vi "GearRectangleCompare.vi"(6 "Line Border":cluster{"Top":dbl, "Bottom":dbl}={"Top"=6.0, "Bottom"=1.0}, 9 "Second":dbl[](array[numeric]), 11 "First":dbl[](array[numeric])) -> (0 "Rect":T1, 1 "Line":T1, 3 "Scores":T2)   [LabVIEW 2016]
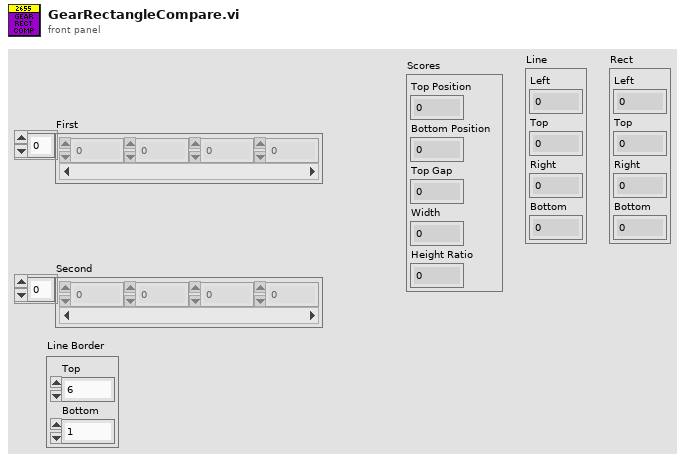
[diagram p1: front panel]
types:
  T1 = cluster{"Left":dbl, "Top":dbl, "Right":dbl, "Bottom":dbl}
  T2 = cluster{"Top Position":dbl, "Bottom Position":dbl, "Top Gap":dbl, "Width":dbl, "Height Ratio":dbl}
  T3 = cluster{"Top Position":dbl, "Bottom Position":dbl, "Left Gap":dbl, "Width":dbl}
  T4 = cluster{"Top Position":dbl, "Bottom Position":dbl, "Left Gap":dbl, "Width":dbl, "Height Ratio":dbl}
  T5 = cluster{"[0]":dbl, "[1]":dbl, "[2]":dbl, "[3]":dbl}
  T6 = cluster{"Top Position":dbl, "Top Position":dbl, "Top Position":dbl, "Top Position":dbl}
  T7 = cluster{"upper limit":dbl, "upper limit":dbl, "upper limit":dbl, "upper limit":dbl, "upper limit":dbl}
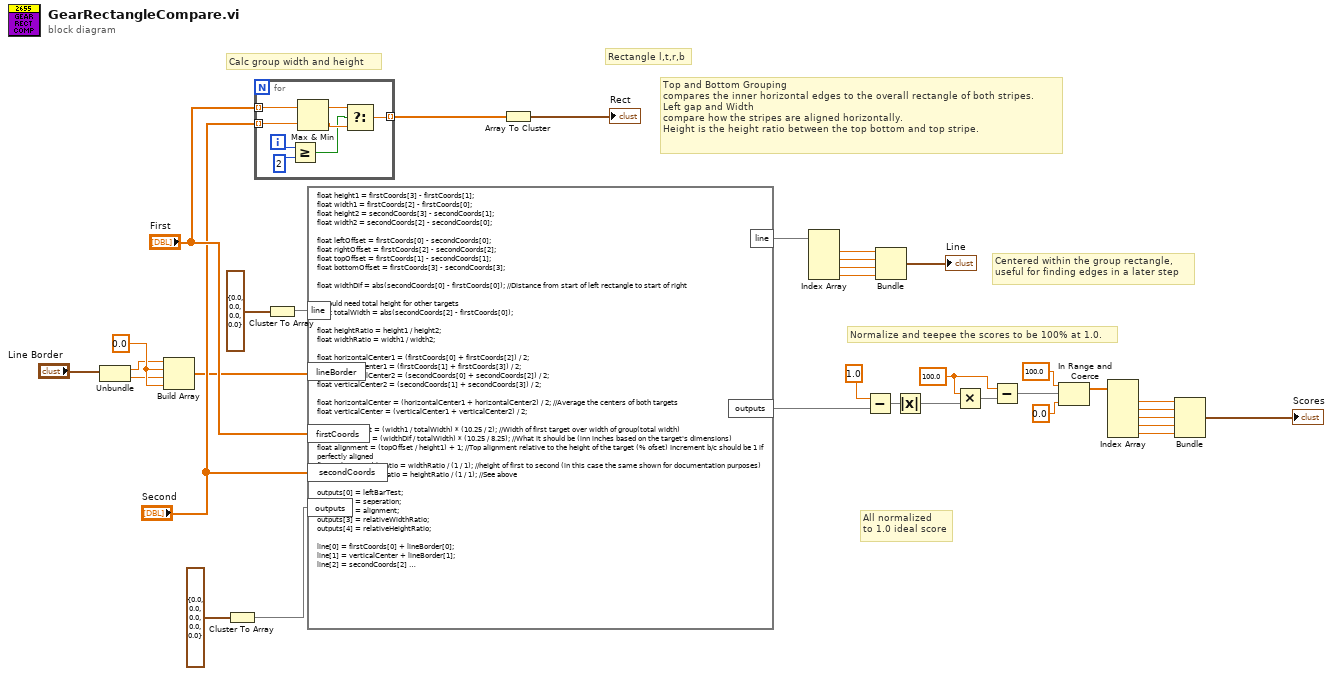
[diagram p0: block diagram]
diagram:
  w3 = 0.0 ("element")
  w31 = 100.0 ("x/y")
  # "Centered within the group rectangle,\nuseful for finding edges in a later step"
  # "All normalized\nto 1.0 ideal score"
  # "Normalize and teepee the scores to be 100% at 1.0."
  # "Top and Bottom Grouping\ncompares the inner horizontal edges to the overall rectangle of both stripes.\nLeft gap and Width\ncompare how the stripes are aligned horizontally.\nHeight is the height ratio between the top bottom and top stripe."
  # "Calc group width and height"
  # "Rectangle l,t,r,b"
  n1 = Unbundle("Line Border") -> ("Top"=w2:dbl, "Bottom"=w1:dbl)
  n2 = Build Array(w2, w3, w1, w3) -> (w4:dbl[])
  n3 = Cluster To Array(cluster=T4 {"Top Position"=0.0, "Bottom Position"=0.0, "Left Gap"=0.0, "Width"=0.0, "Height Ratio"=0.0} ("Scores 2")) -> (array=w14:dbl[])
  n4 = for {
    tunnel: "First" -> [w43] mode=indexing
    tunnel: "Second" -> [w42] mode=indexing
    tunnel: [w36] -> w35 mode=indexing
    i -> [w40]
    n5 = Greater Or Equal?(x=w40, y=2) -> (x >= y?=w37:bool)
    n6 = Max & Min(x=w43, y=w42) -> (max(x,y)=w39:dbl, min(x,y)=w38:dbl)
    n7 = Select(t=w39, s=w37, f=w38) -> (s? t:f=w36:dbl)
  }
  n8 = Cluster To Array(cluster=T3 {"Top Position"=0.0, "Bottom Position"=0.0, "Left Gap"=0.0, "Width"=0.0} ("Scores 2")) -> (array=w12:dbl[])
  n9 = formula code="float height1 = firstCoords[3] - firstCoords[1];\nfloat width1 = firstCoords[2] - firstCoords[0];\nfloat height2 = secondCoords[3] - secondCoords[1];\nfloat width2 = secondCoords[2] - secondCoords[0];\n\nfloat leftOffset = firstCoords[0] - secondCoords[0];\nfloat rightOffset = firstCoords[2] - secondCoords[2];\nfloat topOffset = firstCoords[1] - secondCoords[1];\nfloat bottomOffset = firstCoords[3] - secondCoords[3];\n\t\nfloat widthDif = abs(secondCoords[0] - firstCoords[0]); //Distance from start of left rectangle to start of right\n\t\n//Would need total height for other targets\nfloat totalWidth = abs(secondCoords[2] - firstCoords[0]);\n\t\nfloat heightRatio = height1 / height2;\nfloat widthRatio = width1 / width2;\n\nfloat horizontalCenter1 = (firstCoords[0] + firstCoords[2]) / 2;\nfloat verticalCenter1 = (firstCoords[1] + firstCoords[3]) / 2;\nfloat horizontalCenter2 = (secondCoords[0] + secondCoords[2]) / 2;\nfloat verticalCenter2 = (secondCoords[1] + secondCoords[3]) / 2;\n\nfloat horizontalCenter = (horizontalCenter1 + horizontalCenter2) / 2; //Average the centers of both targets\nfloat verticalCenter = (verticalCenter1 + verticalCenter2) / 2;\n\t\t\nfloat leftBarTest = (width1 / totalWidth) * (10.25 / 2); //Width of first target over width of group(total width)\nfloat seperation = (widthDif / totalWidth) * (10.25 / 8.25); //What it should be (inn inches based on the target's dimensions)\nfloat alignment = (topOffset / height1) + 1; //Top alignment relative to the height of the target (% ofset) Increment b/c should be 1 if perfectly aligned\nfloat relativeWidthRatio = widthRatio / (1 / 1); //height of first to second (in this case the same shown for documentation purposes)\nfloat relativeHeightRatio = heightRatio / (1 / 1); //See above\n\t\t\t\t\noutputs[0] = leftBarTest;\noutputs[1] = seperation;\noutputs[2] = alignment;\noutputs[3] = relativeWidthRatio;\noutputs[4] = relativeHeightRatio;\n\t\t\nline[0] = firstCoords[0] + lineBorder[0];\nline[1] = verticalCenter + lineBorder[1];\nline[2] = secondCoords[2] - lineBorder[2];\nline[3] = verticalCenter - lineBorder[3];"("firstCoords"="First", "secondCoords"="Second", "outputs"=w14, "line"=w12, "lineBorder"=w4) -> ("outputs"=w23:dbl[], "line"=w7:dbl[])
  n10 = Array To Cluster(array=w35) -> (cluster=→"Rect":T5)
  n11 = Index Array(array=w7) -> (element #1=w11:dbl, element #2=w10:dbl, element #3=w9:dbl, element #4=w8:dbl)  [unwired: 4 in]
  n12 = Subtract(x=1.0 ("y"), y=w23) -> (x-y=w29:dbl[])
  n13 = Bundle("Top Position"=w11, "Top Position"=w10, "Top Position"=w9, "Top Position"=w8) -> (→"Line":T6)  [unwired: 1 in]
  n14 = Absolute Value(x=w29) -> (abs(x)=w32:dbl[])
  n15 = Multiply(x=w31, y=w32) -> (x*y=w33:dbl[])
  n16 = Subtract(x=w31, y=w33) -> (x-y=w28:dbl[])
  n17 = In Range and Coerce(upper limit=100.0, x=w28, lower limit=0.0) -> (coerced(x)=w22:dbl[])  [unwired: 1 out]
  n18 = Index Array(array=w22) -> (element #1=w21:dbl, element #2=w20:dbl, element #3=w19:dbl, element #4=w18:dbl, element #5=w17:dbl)  [unwired: 5 in]
  n19 = Bundle("upper limit"=w21, "upper limit"=w20, "upper limit"=w19, "upper limit"=w18, "upper limit"=w17) -> (→"Scores":T7)  [unwired: 1 in]
